vi "Error Generator.vi"(7 "Details":string, 10 "error in (no error)":errorcluster, 11 "Error selector":T1) -> (2 "error out":errorcluster)   [LabVIEW 2020, in "UI_Actor.lvlib" / "UI_Actor.lvclass"]
uses:
  UI_Actor.lvclass
  ctl_ErrorSelector.ctl
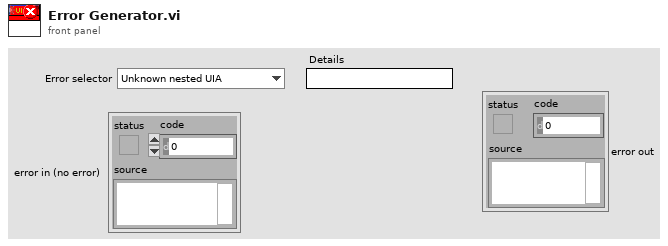
[diagram p1: front panel]
types:
  T1 = typedef "ctl_ErrorSelector.ctl" = enum16{"Unknown nested UIA", "Unsupported type"}
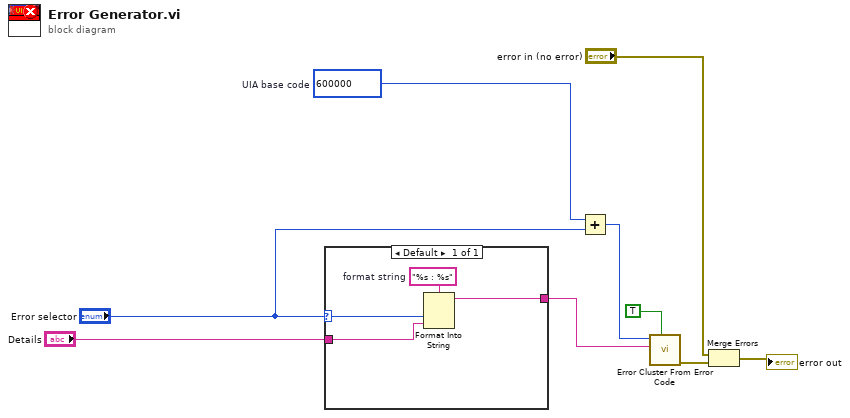
[diagram p0: block diagram]
diagram:
  w9 = 600000  # UIA base code
  n1 = case shown="Default" "Error selector" {
    selector: "Error selector" -> [w13]
    tunnel: [w12] -> w6
    tunnel: "Details" -> [w10]
    frame Default {
      w11 = "%s : %s"  # format string
      n2 = Format Into String(format string=w11, w13, w10) -> (resulting string=w12:string)  [unwired: 2 in, 1 out]
    }
  }
  n3 = Add(x=w9, y="Error selector") -> (x+y=w5:i32)
  n4 = call <vilib>:"Error Cluster From Error Code.vi"("show call chain? (False)"=TRUE, "error message (\"\")"=w6, "error code (0)"=w5) -> ("error out"=w3:errorcluster)  [unwired: 6 in]
  n5 = Merge Errors("error in (no error)", w3) -> (→"error out":errorcluster)
